vi "Run.vi"(8 "error in (no error)":errorcluster, 11 "Opctics in":refnum<class "Opt_Continuous.lvclass">) -> (0 "error out":errorcluster, 3 "Opt_Continuous out":refnum<class "Opt_Continuous.lvclass">)   [LabVIEW 2018, in "Opt_Continuous.lvclass"]
uses:
  Opt_Continuous.lvclass
  C:/Users/devstaff/sparc4/s4gui/Versao ZeroMQ REQ-REP/SPARC4_GUI -v1.0.0 - 20250122_ICS-JSON/Device/Optics/Optics.lvclass
  Optics.lvclass/Optics.ctl
  Optics.lvclass
  StateMachine/State Machine.lvclass
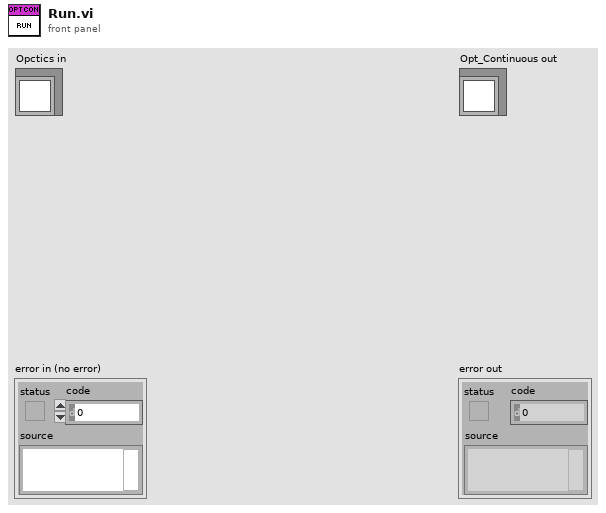
[diagram p1: front panel]
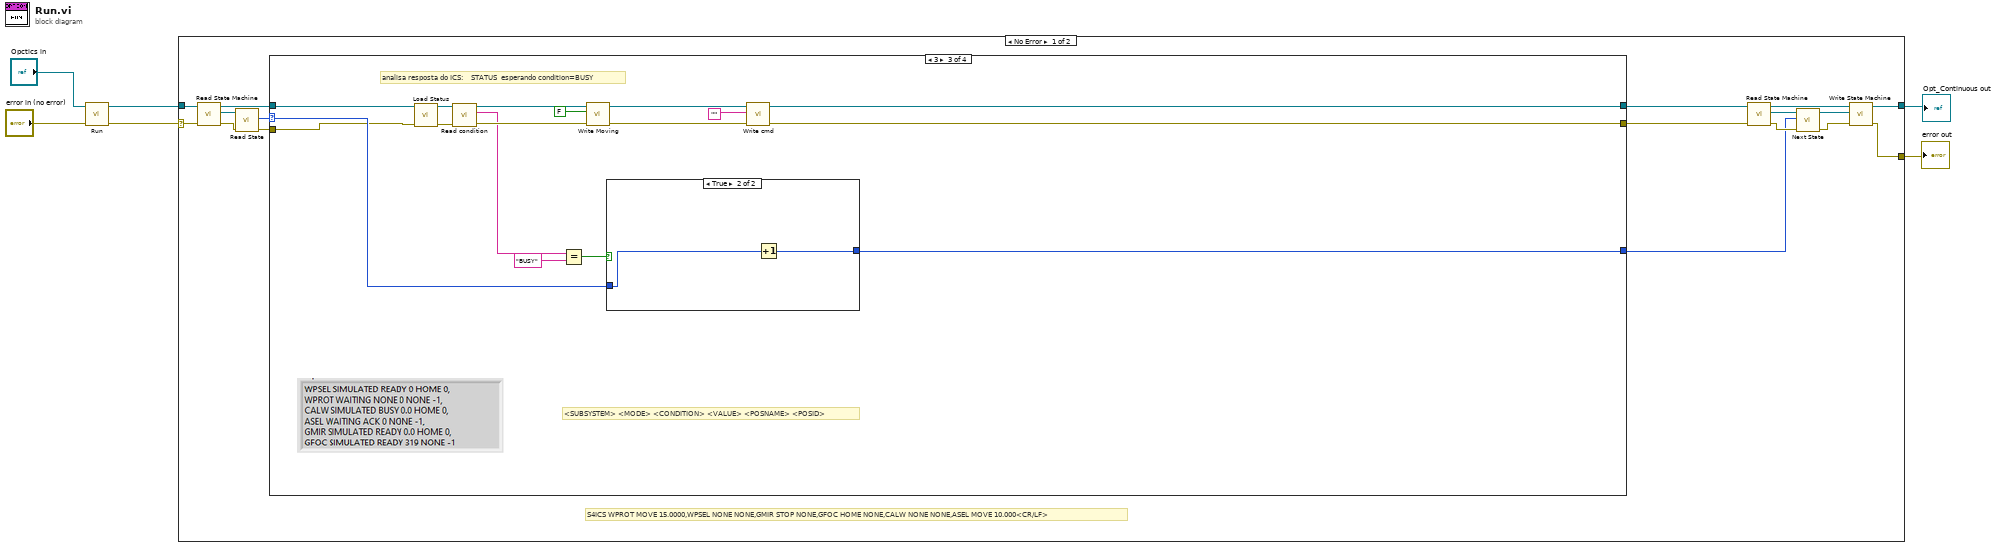
[diagram p0: block diagram]
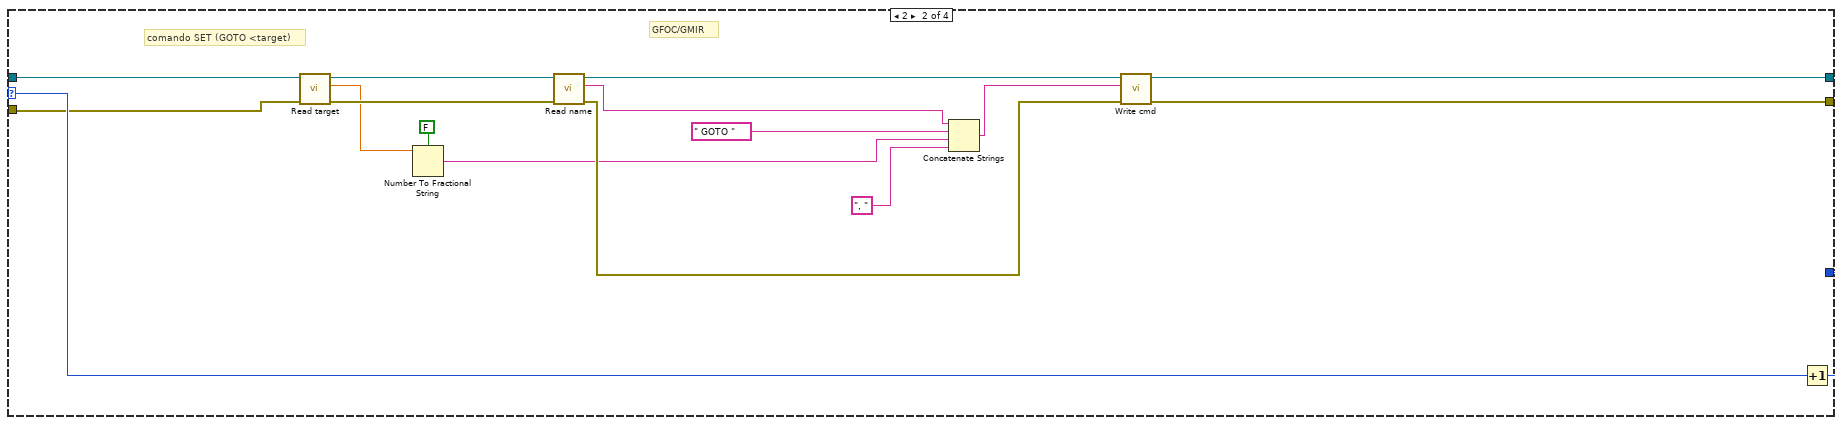
[diagram p3: hidden frame]
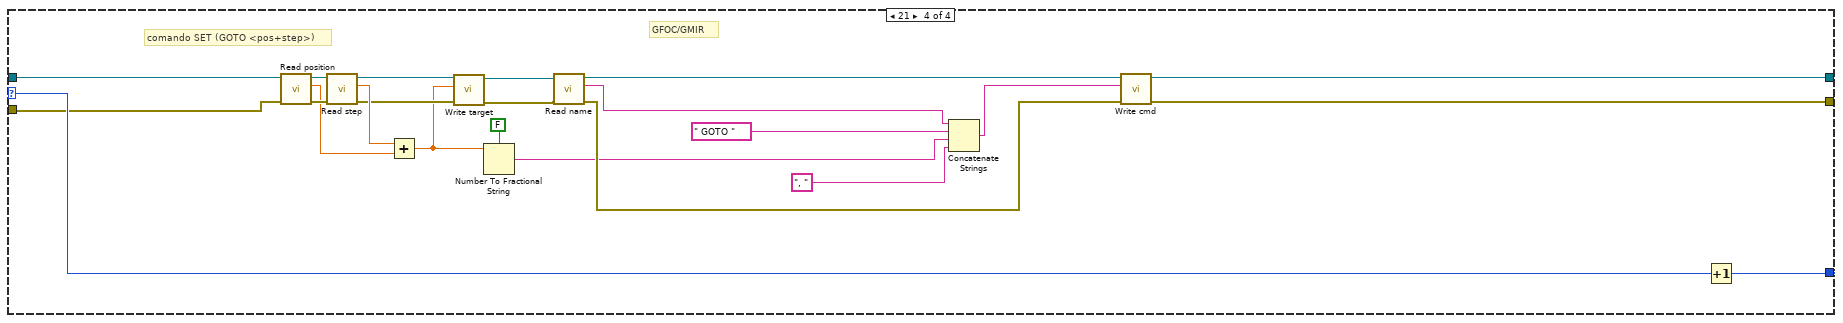
[diagram p5: hidden frame]
diagram:
  n1 = call-parent "Run.vi"("error in (no error)"="error in (no error)", "Opctics in"="Opctics in") -> ("error out"=w4:errorcluster, "Optics out"=w3:refnum<class "Opt_Continuous.lvclass">)  [unwired: 8 in]
  n2 = case shown="No Error" w4 {
    selector: w4 -> [w22 w88]
    tunnel: [w7 w88] -> w1
    tunnel: [w12 w87] -> w2
    tunnel: w3 -> [w23 w87]
    frame No Error {
      # "S4ICS WPROT MOVE 15.0000,WPSEL NONE NONE,GMIR STOP NONE,GFOC HOME NONE,CALW NONE NONE,ASEL MOVE 10.000<CR/LF>"
      n3 = call-dynamic "Read State Machine.vi"("error in (no error)"=w22, "Device in"=w23) -> ("error out"=w19:errorcluster, "State Machine.lvclass"=w21:refnum<class "State Machine.lvclass">, "Device out"=w17:refnum<class "Opt_Continuous.lvclass">)  [unwired: 7 in]
      n4 = call-dynamic "Read State.vi"("error in (no error)"=w19, "State Machine in"=w21) -> ("error out"=w18:errorcluster, "State"=w20:i32)  [unwired: 7 in, 1 out]
      n5 = case shown="3" w20 {
        selector: w20 -> [w26 w39 w59 w82]
        tunnel: w18 -> [w24 w36 w51 w79]
        tunnel: [w24 w42 w57 w85] -> w8
        tunnel: w17 -> [w25 w37 w52 w80]
        tunnel: [w25 w43 w58 w86] -> w15
        tunnel: [w26 w40 w56 w83] -> w9
        frame Default {
        }
        frame 2 {
          # "GFOC/GMIR"
          # "comando SET (GOTO <target)"
          n6 = call "Read target.vi"("error in (no error)"=w36, "Optics in"=w37) -> ("error out"=w34:errorcluster, "target"=w30:dbl, "Optics out"=w32:refnum<class "Opt_Continuous.lvclass">)  [unwired: 7 in]
          n7 = Number To Fractional String(use system decimal point (T)=FALSE, number=w30) -> (F-format string=w29:string)  [unwired: 2 in]
          n8 = call "Read name.vi"("error in (no error)"=w34, "Optics in"=w32) -> ("error out"=w33:errorcluster, "name"=w35:string, "Optics out"=w31:refnum<class "Opt_Continuous.lvclass">)  [unwired: 7 in]
          n9 = Concatenate Strings(w35, " GOTO " ("string"), w29, ", ") -> (w41:string)
          n10 = call-dynamic "Write cmd.vi"("error in (no error)"=w33, "cmd"=w41, "Device in"=w31) -> ("error out"=w42:errorcluster, "Device out"=w43:refnum<class "Opt_Continuous.lvclass">)  [unwired: 7 in]
          n11 = Increment(x=w39) -> (x+1=w40:i32)
        }
        frame 3 {
          # "<SUBSYSTEM> <MODE> <CONDITION> <VALUE> <POSNAME> <POSID>"
          # "analisa resposta do ICS:    STATUS  esperando condition=BUSY"
          n12 = call-dynamic "Load Status.vi"("error in (no error)"=w51, "Optics in"=w52) -> ("error out"=w49:errorcluster, "Optics out"=w50:refnum<class "Opt_Continuous.lvclass">)  [unwired: 8 in]
          n13 = call "Read condition.vi"("error in (no error)"=w49, "Optics in"=w50) -> ("error out"=w48:errorcluster, "condition"=w46:string, "Optics out"=w45:refnum<class "Opt_Continuous.lvclass">)  [unwired: 7 in]
          n14 = Equal?(x=w46, y="BUSY") -> (x = y?=w54:bool)
          n15 = call-dynamic "Write Moving.vi"("error in (no error)"=w48, "Moving"=FALSE, "Optics in"=w45) -> ("error out"=w47:errorcluster, "Optics out"=w44:refnum<class "Opt_Continuous.lvclass">)  [unwired: 7 in]
          n16 = case shown="True" w54 {
            tunnel: [w61 w62] -> w56
            tunnel: w59 -> [w61 w63]
            frame False {
            }
            frame True {
              n17 = Increment(x=w63) -> (x+1=w62:i32)
            }
          }
          n18 = call-dynamic "Write cmd.vi"("error in (no error)"=w47, "cmd"="", "Device in"=w44) -> ("error out"=w57:errorcluster, "Device out"=w58:refnum<class "Opt_Continuous.lvclass">)  [unwired: 7 in]
        }
        frame 21 {
          # "GFOC/GMIR"
          # "comando SET (GOTO <pos+step>)"
          n19 = call "Read position.vi"("error in (no error)"=w79, "Optics in"=w80) -> ("error out"=w72:errorcluster, "position"=w70:dbl, "Optics out"=w73:refnum<class "Opt_Continuous.lvclass">)  [unwired: 7 in]
          n20 = call-dynamic "Read step.vi"("error in (no error)"=w72, "Optics in"=w73) -> ("error out"=w67:errorcluster, "step"=w71:dbl, "Optics out"=w69:refnum<class "Opt_Continuous.lvclass">)  [unwired: 7 in]
          n21 = Add(x=w71, y=w70) -> (x+y=w65:dbl)
          n22 = call "Write target.vi"("error in (no error)"=w67, "target"=w65, "Optics in"=w69) -> ("error out"=w66:errorcluster, "Optics out"=w68:refnum<class "Opt_Continuous.lvclass">)  [unwired: 7 in]
          n23 = Number To Fractional String(use system decimal point (T)=FALSE, number=w65) -> (F-format string=w75:string)  [unwired: 2 in]
          n24 = call "Read name.vi"("error in (no error)"=w66, "Optics in"=w68) -> ("error out"=w77:errorcluster, "name"=w78:string, "Optics out"=w76:refnum<class "Opt_Continuous.lvclass">)  [unwired: 7 in]
          n25 = Concatenate Strings(w78, " GOTO " ("string"), w75, ", ") -> (w84:string)
          n26 = call-dynamic "Write cmd.vi"("error in (no error)"=w77, "cmd"=w84, "Device in"=w76) -> ("error out"=w85:errorcluster, "Device out"=w86:refnum<class "Opt_Continuous.lvclass">)  [unwired: 7 in]
          n27 = Increment(x=w82) -> (x+1=w83:i32)
        }
      }
      n28 = call-dynamic "Read State Machine.vi"("error in (no error)"=w8, "Device in"=w15) -> ("error out"=w11:errorcluster, "State Machine.lvclass"=w14:refnum<class "State Machine.lvclass">, "Device out"=w13:refnum<class "Opt_Continuous.lvclass">)  [unwired: 7 in]
      n29 = call "Next State.vi"("error in (no error)"=w11, "New_State"=w9, "State Machine in"=w14) -> ("error out"=w10:errorcluster, "State Machine out"=w16:refnum<class "State Machine.lvclass">)  [unwired: 7 in]
      n30 = call-dynamic "Write State Machine.vi"("error in (no error)"=w10, "State Machine.lvclass"=w16, "Device in"=w13) -> ("error out"=w7:errorcluster, "Device out"=w12:refnum<class "Opt_Continuous.lvclass">)  [unwired: 7 in]
    }
    frame Error {
    }
  }
  "error out" <- w1
  "Opt_Continuous out" <- w2
